vi "Get pin Status.vi"(8 "error in (no error)":errorcluster, 9 "Pin 2":dbl, 10 "Puerto":dbl, 11 "Cypress in":refnum<class "Cypress.lvclass">) -> (0 "error out":errorcluster, 3 "Cypress out":refnum<class "Cypress.lvclass">)   [LabVIEW 2020, in "Cypress.lvclass"]
uses:
  Cypress.lvclass
  8b774dff-84e1-4193-8858-12d827949e44.vi
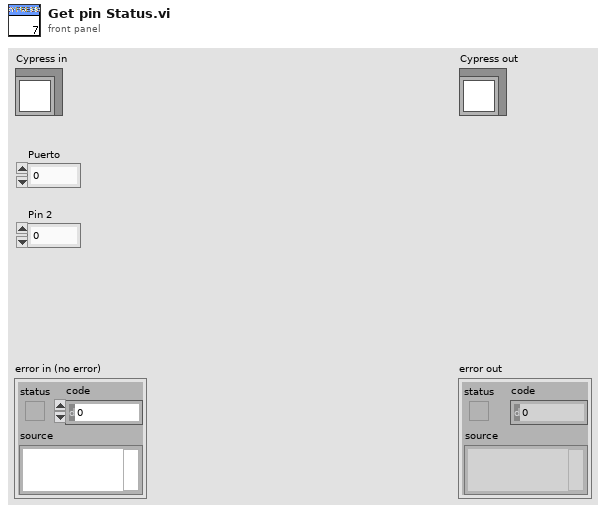
[diagram p1: front panel]
types:
  T1 = typedef "Serial Device.lvclass/serial device brand.ctl" = string
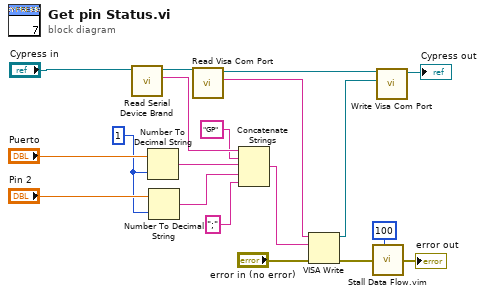
[diagram p0: block diagram]
diagram:
  w13 = i16 1 ("width (-)")
  n1 = call-dynamic "Read Serial Device Brand.vi"("Serial Device in"="Cypress in") -> ("Serial Device Brand"=w12:T1, "Serial Device out"=w18:refnum<class "Cypress.lvclass">)  [unwired: 8 in, 1 out]
  n2 = Number To Decimal String(number="Puerto", width (-)=w13) -> (decimal integer string=w10:string)
  n3 = Number To Decimal String(number="Pin 2", width (-)=w13) -> (decimal integer string=w9:string)
  n4 = call-dynamic "Read Visa Com Port.vi"("Serial Device in"=w18) -> ("Visa Com Port"=w7:string, "Serial Device out"=w17:refnum<class "Cypress.lvclass">)  [unwired: 8 in, 1 out]
  n5 = Concatenate Strings(w12, "GP" ("string"), w10, w9, ";" ("string")) -> (w5:string)
  n6 = VISA Write(VISA resource name=w7, write buffer=w5, error in (no error)="error in (no error)") -> (VISA resource name out=w6:refnum<visa-resource-name>, error out=w3:errorcluster)  [unwired: 1 out]
  n7 = call "Stall Data Flow.vim"("value in"=w3, "milliseconds to wait"=u32 100) -> ("value out"=→"error out":errorcluster)  [unwired: 1 out]
  n8 = call-dynamic "Write Visa Com Port.vi"("Visa Com Port"=w6, "Serial Device in"=w17) -> ("Serial Device out"=→"Cypress out":refnum<class "Cypress.lvclass">)  [unwired: 8 in, 1 out]
